vi "SS Write Data Q.vi"(8 "error in (no error)":errorcluster, 10 "Data Q":refnum<queue>, 11 "Subsystem Class in":refnum<class "Subsystem Class.lvclass">) -> (0 "error out":errorcluster, 3 "Subsystem Class out":refnum<class "Subsystem Class.lvclass">)   [LabVIEW 2024, in "Subsystem Class.lvclass"]
uses:
  Subsystem Class.lvclass
  SS cluster Data Queue type.ctl
  Subsystem Class.lvclass/Subsystem Class.ctl
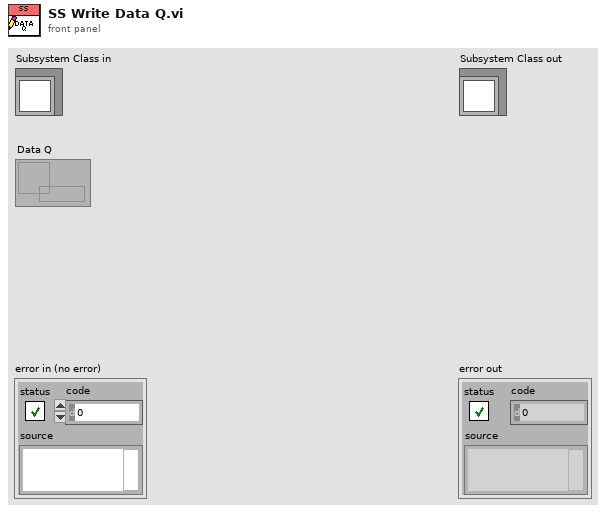
[diagram p1: front panel]
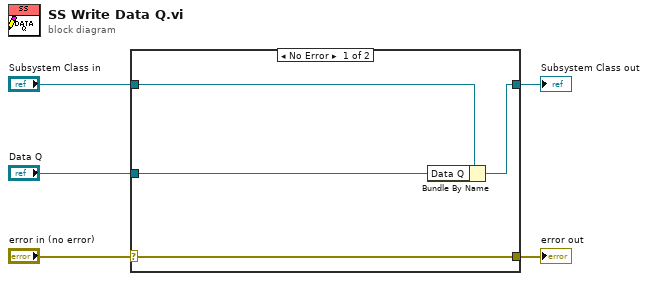
[diagram p0: block diagram]
diagram:
  n1 = case shown="No Error" "error in (no error)" {
    selector: "error in (no error)" -> [w9 w10]
    tunnel: [w9 w10] -> w4
    tunnel: [w7 w11] -> w2
    tunnel: "Subsystem Class in" -> [w8 w11]
    tunnel: "Data Q" -> [w6 _]
    frame No Error {
      n2 = Bundle By Name(cluster=w8, "Data Q"=w6) -> (w7:refnum<class "Subsystem Class.lvclass">)
    }
    frame Error {
    }
  }
  "error out" <- w4
  "Subsystem Class out" <- w2
